vi "MB Decode Data.vi"(8 "error in (no error)":errorcluster, 10 "Response MDU":cluster{"Function Code":u8, "Data":u8[]}={"Function Code"=1, "Data"=[]} {"Function Code" items=["Read Coils"=1, "Read Discrete Inputs"=2, "Read Holding Registers"=3, "Read Input Registers"=4, "Write Single Coil"=5, "Write Single Register"=6, "Read Exception Status"=7, "Write Multiple Coils"=15, "Write Multiple Registers"=16]; "Data" format="%.0x"}, 11 "Request MDU":cluster{"Function Code":u8, "Data":u8[]}={"Function Code"=1, "Data"=[]} {"Function Code" items=["Read Coils"=1, "Read Discrete Inputs"=2, "Read Holding Registers"=3, "Read Input Registers"=4, "Write Single Coil"=5, "Write Single Register"=6, "Read Exception Status"=7, "Write Multiple Coils"=15, "Write Multiple Registers"=16]; "Data" format="%.0x"}) -> (0 "error out":errorcluster, 2 "Discrete":bool[](array[boolean]), 3 "Registers":u16[](array[numeric]))   [LabVIEW 2017]
panel:
  # "VI Name: MB Decode Data.vi\nPurpose: Decodes a MODBUS Data Unit to return the actual values of the registers read to the user.\nReentrant  VI"
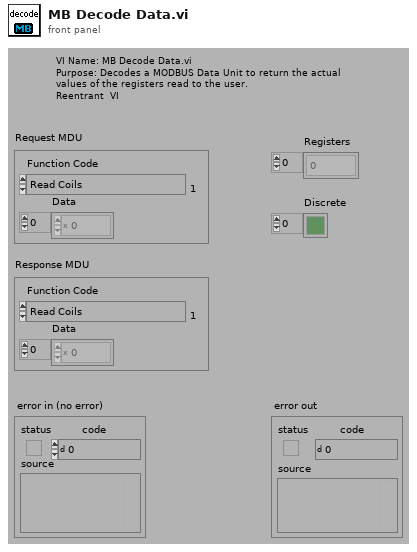
[diagram p1: front panel]
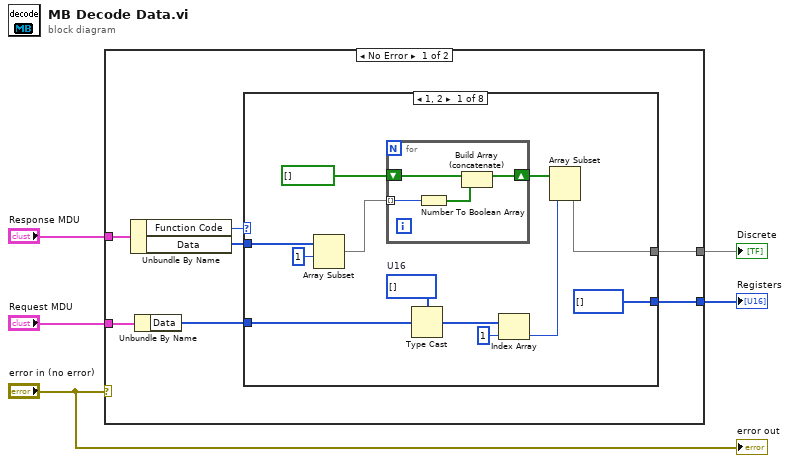
[diagram p0: block diagram]
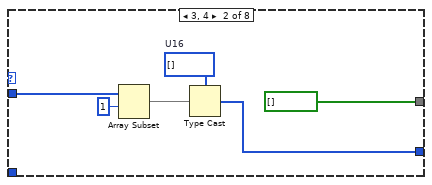
[diagram p2: hidden frame]
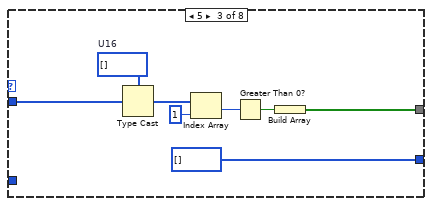
[diagram p3: hidden frame]
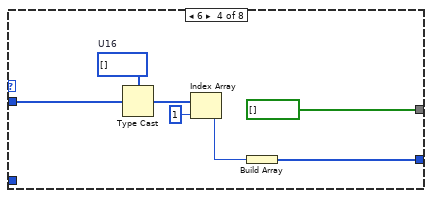
[diagram p4: hidden frame]
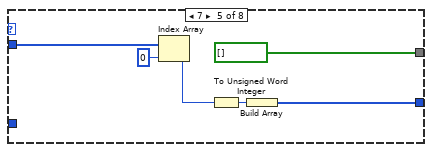
[diagram p5: hidden frame]
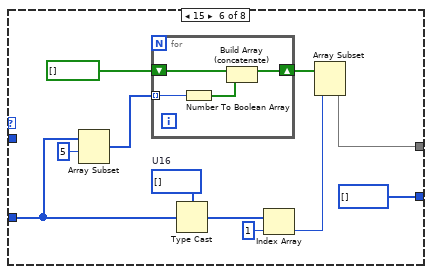
[diagram p6: hidden frame]
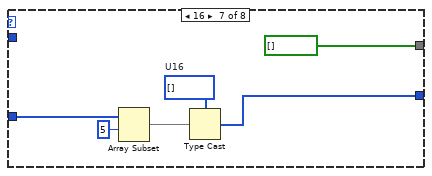
[diagram p7: hidden frame]
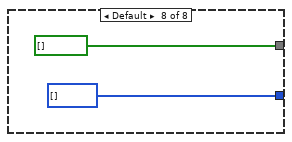
[diagram p8: hidden frame]
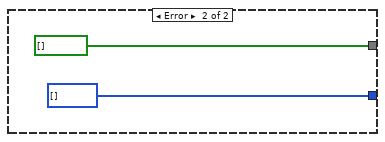
[diagram p9: hidden frame]
diagram:
  n1 = case shown="No Error" "error in (no error)" {
    tunnel: "Response MDU" -> [w12 _]
    tunnel: [w9 bool[] []] -> w4
    tunnel: [w8 u16[] [] ("U16")] -> w3
    tunnel: "Request MDU" -> [w7 _]
    frame No Error {
      n2 = Unbundle By Name(w12) -> ("Function Code"=w11:u8, "Data"=w10:u8[])
      n3 = Unbundle By Name(w7) -> ("Data"=w6:u8[])
      n4 = case shown="1, 2" w11 {
        tunnel: w10 -> [w24 w34 w36 w47 w51 _ _ _]
        tunnel: [w13 bool[] [] w38 bool[] [] bool[] [] w57 bool[] [] bool[] []] -> w9
        tunnel: [u16[] [] w30 u16[] [] w44 w53 u16[] [] w73 u16[] [] ("U16")] -> w8
        tunnel: w6 -> [w18 _ _ _ _ w56 w71 _]
        frame 1, 2 {
          w17 = u16[] []  # U16
          n5 = Array Subset(array=w24, index=1) -> (w20:u8[])  [unwired: 1 in]
          n6 = for {
            shift-right: [w27] -> w19
            shift-left: bool[] [] -> [w28]
            tunnel: w20 -> [w26] mode=indexing
            n7 = Number To Boolean Array(number=w26) -> (Boolean array=w25:bool[])
            n8 = Build Array (concatenate)(w28, w25) -> (w27:bool[])
          }
          n9 = Type Cast(type=w17, x=w18) -> (*(type *) &x=w16:u16[])
          n10 = Index Array(array=w16, index=1) -> (element=w14:u16)
          n11 = Array Subset(array=w19, length=w14) -> (w13:bool[])  [unwired: 1 in]
        }
        frame 3, 4 {
          w31 = u16[] []  # U16
          n12 = Array Subset(array=w34, index=1) -> (w32:u8[])  [unwired: 1 in]
          n13 = Type Cast(type=w31, x=w32) -> (*(type *) &x=w30:u16[])
        }
        frame 5 {
          w37 = u16[] []  # U16
          n14 = Type Cast(type=w37, x=w36) -> (*(type *) &x=w35:u16[])
          n15 = Index Array(array=w35, index=1) -> (element=w40:u16)
          n16 = Greater Than 0?(x=w40) -> (x > 0?=w39:bool)
          n17 = Build Array(w39) -> (w38:bool[])
        }
        frame 6 {
          w48 = u16[] []  # U16
          n18 = Type Cast(type=w48, x=w47) -> (*(type *) &x=w46:u16[])
          n19 = Index Array(array=w46, index=1) -> (element=w45:u16)
          n20 = Build Array(w45) -> (w44:u16[])
        }
        frame 7 {
          n21 = Index Array(array=w51, index=0) -> (element=w54:u8)
          n22 = To Unsigned Word Integer(number=w54) -> (unsigned 16bit integer=w50:u16)
          n23 = Build Array(w50) -> (w53:u16[])
        }
        frame 15 {
          w61 = u16[] []  # U16
          n24 = Array Subset(array=w56, index=5) -> (w63:u8[])  [unwired: 1 in]
          n25 = for {
            shift-right: [w69] -> w62
            shift-left: bool[] [] -> [w70]
            tunnel: w63 -> [w67] mode=indexing
            n26 = Number To Boolean Array(number=w67) -> (Boolean array=w68:bool[])
            n27 = Build Array (concatenate)(w70, w68) -> (w69:bool[])
          }
          n28 = Type Cast(type=w61, x=w56) -> (*(type *) &x=w60:u16[])
          n29 = Index Array(array=w60, index=1) -> (element=w58:u16)
          n30 = Array Subset(array=w62, length=w58) -> (w57:bool[])  [unwired: 1 in]
        }
        frame 16 {
          w74 = u16[] []  # U16
          n31 = Array Subset(array=w71, index=5) -> (w75:u8[])  [unwired: 1 in]
          n32 = Type Cast(type=w74, x=w75) -> (*(type *) &x=w73:u16[])
        }
        frame Default {
        }
      }
    }
    frame Error {
    }
  }
  "Registers" <- w3
  "Discrete" <- w4
  "error out" <- "error in (no error)"
